vi "Update Status Message for Test.vi"(11 "Parallel Test in":refnum<class "Parallel Test.lvclass">) -> ()   [LabVIEW 2015, in "Parallel Test.lvclass"]
uses:
  Parallel Test.lvclass
  Test Class/Test Class.lvclass
  Classes/Application/Class/Application.lvclass
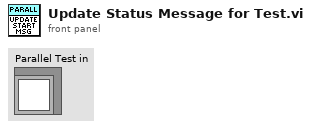
[diagram p1: front panel]
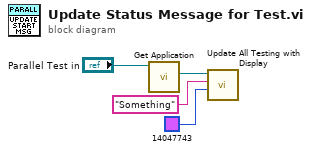
[diagram p0: block diagram]
diagram:
  n1 = call "Get Application.vi"("Test Class in"="Parallel Test in") -> ("Application.lvlib:Application.lvclass"=w4:refnum<class "Application.lvclass">)  [unwired: 9 in, 1 out]
  n2 = call "Update All Testing with Display.vi"("BG Color"=u32 14047743, "Message ('')"="Something", "Application in"=w4) -> ()  [unwired: 7 in, 2 out]
